vi "Guitar String.vi"() -> ()   [LabVIEW 2012]
uses:
  <vilib>/ptbypt/NI_PtbyPt.lvlib
panel:
  in  "stop":bool
  in  "P":i32(slide) scale=0.0..10.0
  out "Waveform Graph":waveform(dbl)(graph)
  in  "N":i32(slide) scale=0.0..10.0
  in  "a":dbl(slide) scale=-1.0..1.0
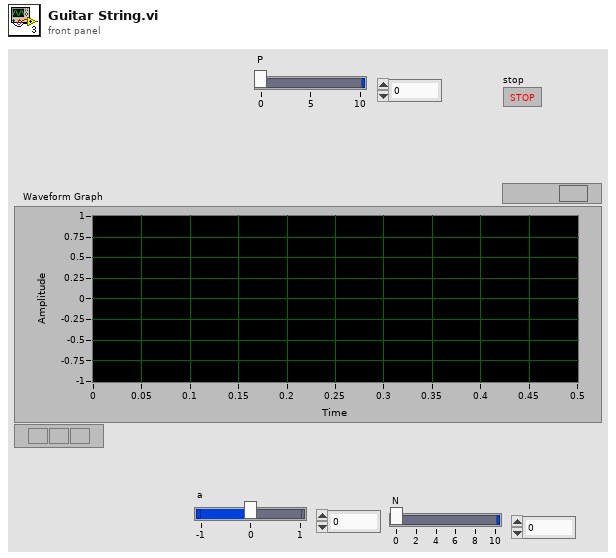
[diagram p1: front panel]
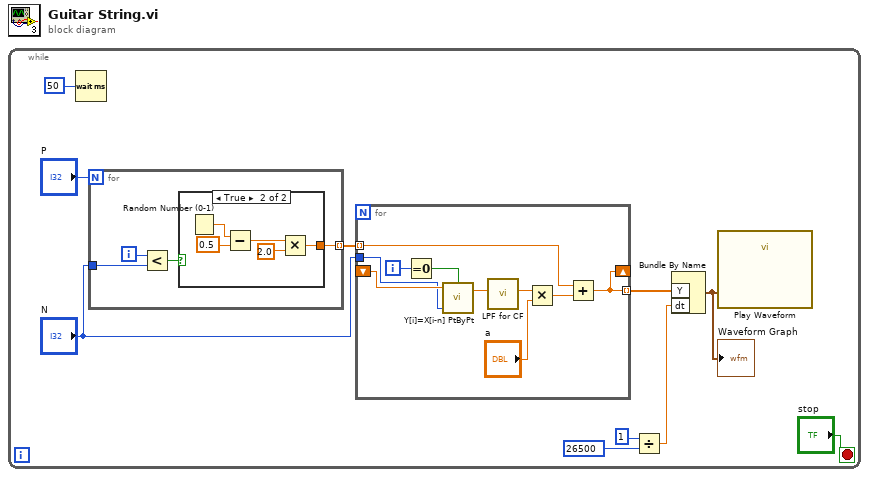
[diagram p0: block diagram]
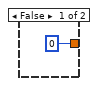
[diagram p2: hidden frame]
diagram:
  n1 = while {
    stop <- "stop" stop-if-true
    n2 = Wait (ms)(milliseconds to wait=50) -> ()  [unwired: 1 out]
    n3 = for {
      N: "P" -> [_]
      tunnel: [w14] -> w9 mode=indexing
      tunnel: "N" -> [w11]
      i -> [w12]
      n4 = Less?(x=w12, y=w11) -> (x < y?=w13:bool)
      n5 = case shown="True" w13 {
        tunnel: [0 w18] -> w14
        frame False {
        }
        frame True {
          n6 = Random Number (0-1)() -> (number: 0 to 1=w20:dbl)
          n7 = Subtract(x=w20, y=0.5) -> (x-y=w17:dbl)
          n8 = Multiply(x=w17, y=2.0) -> (x*y=w18:dbl)
        }
      }
    }
    n9 = for {
      shift-right: [w25] -> _
      shift-left: _ -> [w27]
      tunnel: [w25] -> w7 mode=indexing
      tunnel: w9 -> [w26] mode=indexing
      tunnel: "N" -> [w24]
      i -> [w29]
      n10 = Equal To 0?(x=w29) -> (x = 0?=w28:bool)
      n11 = call <vilib>:"Y[i]=X[i-n] PtByPt.vi"("initialize"=w28, "shifts: n"=w24, "x"=w27) -> ("shifted x"=w22:dbl)  [unwired: 1 in, 1 out]
      n12 = call "LPF for CF.vi"("Numeric"=w22) -> ("Numeric 2"=w21:dbl)  [unwired: 10 in]
      n13 = Multiply(x=w21, y="a") -> (x*y=w30:dbl)
      n14 = Add(x=w26, y=w30) -> (x+y=w25:dbl)
    }
    n15 = Divide(x=1, y=26500) -> (x/y=w4:dbl)
    n16 = Bundle By Name("Y"=w7, "dt"=w4) -> (w8:waveform(dbl))  [unwired: 1 in]
    "Waveform Graph" <- w8
    n17 = call "Play Waveform"("Data"=w8) -> ()  [unwired: 18 in, 1 out]
  }
